vi "扫描方向检查.vi"(1 "扫描方向":bool[](array[boolean])) -> (0 "检查通过？":bool)   [LabVIEW 2020]
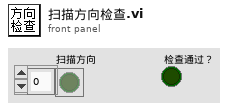
[diagram p1: front panel]
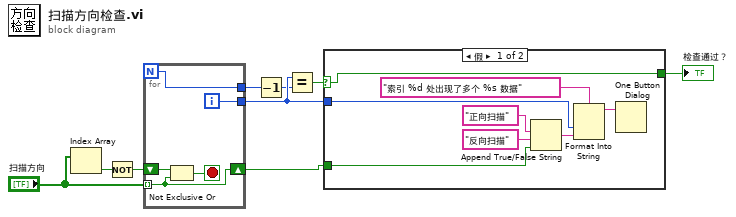
[diagram p0: block diagram]
diagram:
  n1 = Index Array(array="扫描方向") -> (element=w2:bool)  [unwired: 1 in]
  n2 = Not(x=w2) -> (.not. x?=w3:bool)
  n3 = for {
    N -> [w13]
    tunnel: "扫描方向" -> [w10] mode=indexing
    shift-right: [w10] -> w7
    shift-left: w3 -> [w11]
    tunnel: [w13] -> w1
    tunnel: [w12] -> w8
    i -> [w12]
    stop <- w14 stop-if-true
    n4 = Not Exclusive Or(1:w10, 2:w11) -> (0:w14:bool)
  }
  n5 = Decrement(x=w1) -> (x-1=w5:i32)
  n6 = Equal?(x=w8, y=w5) -> (x = y?=w6:bool)
  n7 = case shown="假" w6 {
    selector: w6 -> [w16 w23]
    tunnel: w7 -> [w22 _]
    tunnel: w8 -> [w18 _]
    tunnel: [w16 w23] -> w9
    frame False {
      n8 = Append True/False String(1:w22, 2:"反向扫描" ("假字符串"), 3:"正向扫描" ("真字符串")) -> (0:w19:string)  [unwired: 1 in]
      n9 = Format Into String(format string="索引 %d 处出现了多个 %s 数据" ("格式字符串"), w18, w19) -> (resulting string=w15:string)  [unwired: 2 in, 1 out]
      n10 = One Button Dialog(message=w15) -> ()  [unwired: 1 in, 1 out]
    }
    frame True {
    }
  }
  "检查通过？" <- w9
